vi "NextUp.vi"   [LabVIEW 2019, in "FloatUtil.lvlib"]
uses:
  FloatUtil.lvlib
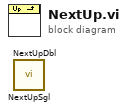
[diagram p0: block diagram]
diagram:
  n1 = call "NextUpSgl.vi"() -> ()  [unwired: 11 in, 1 out]
  n2 = call "NextUpDbl.vi"() -> ()  [unwired: 11 in, 1 out]
